vi "Log Result.vi"(8 "error in (no error)":errorcluster, 10 "tdms file":refnum<k34>, 11 "Find Peaks Result in":refnum<class "Find Peaks Result.lvclass">) -> (0 "error out":errorcluster, 2 "tdms file out":refnum<k34>, 3 "Find Peaks Result out":refnum<class "Find Peaks Result.lvclass">)   [LabVIEW 2015, in "Find Peaks Result.lvclass"]
uses:
  Find Peaks Result.lvclass
  Mag Lab Result.lvclass/Mag Lab Result.ctl
  Find Peaks Result.lvclass/Find Peaks Result.ctl
  Read Group Name.vi
  Read Channel names.vi
  Mag Lab Result.lvclass
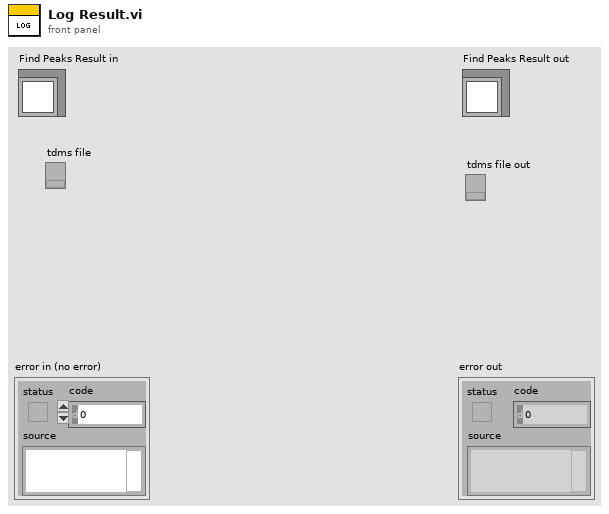
[diagram p1: front panel]
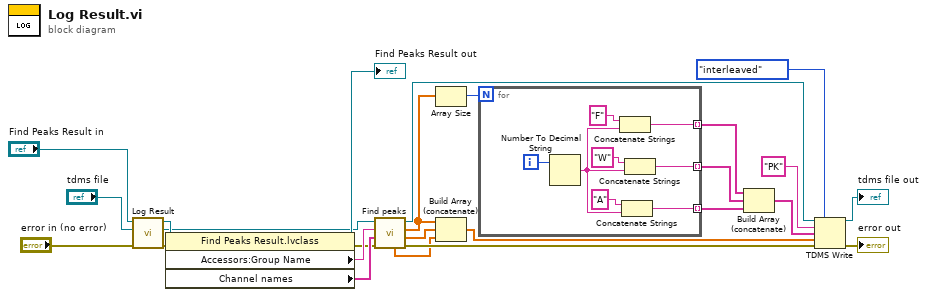
[diagram p0: block diagram]
diagram:
  n1 = call-parent "Log Result.vi"("error in (no error)"="error in (no error)", "tdms file"="tdms file", "Mag Lab Result in"="Find Peaks Result in") -> ("error out"=w5:errorcluster, "tdms file out"=w1:refnum<k34>, "Mag Lab Result out"=w6:refnum<class "Find Peaks Result.lvclass">)  [unwired: 6 in]
  n2 = property class="Find Peaks Result.lvclass"(reference=w6, error in=w5) -> (reference out=→"Find Peaks Result out":refnum<class "Find Peaks Result.lvclass">, error out=w3:errorcluster, "Accessors:Group Name"=w23:string, "Channel names"=w22:string[])
  n3 = call "Find peaks.vi"("Error In"=w3, "Channel names"=w22, "group name"=w23, "tdms file"=w1) -> ("Error Out"=w17:errorcluster, "Width"=w12:dbl[], "Peak F"=w13:dbl[], "tdms file out"=w21:refnum<k34>, "Peak Amplitude"=w11:dbl[])  [unwired: 3 in]
  n4 = Array Size(array=w13) -> (size(s)=w18:i32)
  n5 = Build Array (concatenate)(w13, w12, w11) -> (w9:dbl[])
  n6 = for {
    N: w18 -> [_]
    tunnel: [w28] -> w16 mode=indexing
    tunnel: [w27] -> w15 mode=indexing
    tunnel: [w26] -> w14 mode=indexing
    i -> [w33]
    n7 = Number To Decimal String(number=w33) -> (decimal integer string=w32:string)  [unwired: 1 in]
    n8 = Concatenate Strings("F", w32) -> (w28:string)
    n9 = Concatenate Strings("A", w32) -> (w26:string)
    n10 = Concatenate Strings("W", w32) -> (w27:string)
  }
  n11 = Build Array (concatenate)(w16, w15, w14) -> (w10:string[])
  n12 = TDMS Write(0:w21, 1:enum16{"decimated", "interleaved"}."interleaved" ("data layout (0:decimated)"), 5:"PK", 7:w10, 9:w9, 11:w17) -> (4:→"tdms file out":refnum<k34>, 15:→"error out":errorcluster)  [unwired: 2 out]
